vi "LCP Set Volume Unit.vi"(7 "Prefix":T2=-3 items=["UNIT"=0, "DECI"=-1, "CENTI"=-2, "MILLI"=-3, "MICRO"=-6], 8 "error in (no error)":errorcluster caption="Fehler (Eingang, kein Fehler)", 10 "Volume Unit":T1 items=["LITRES"=68], 11 "Pump Handle":i64) -> (0 "error out":errorcluster caption="Fehler (Ausgang)")   [LabVIEW 2023, in "labbCAN_Pump_API.lvlib"]
doc: "LCP_Func long LCP_CALL LCP_SetVolumeUnit(dev_hdl hPump,\n int Prefix,\n int VolumeUnit);"
uses:
  labbCAN_Pump_API.lvlib
  labbCAN_Bus_API/SiUnitPrefix.ctl
  VolumeUnits.ctl
  labbCAN_Pump_API.dll
  labbCAN_Bus_API/labbCAN_Bus_API.lvlib
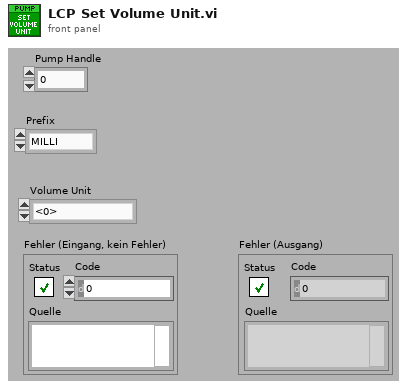
[diagram p1: front panel]
types:
  T1 = typedef "labbCAN_Pump_API.lvlib/VolumeUnits.ctl" = i32
  T2 = typedef "labbCAN_Bus_API.lvlib/SiUnitPrefix.ctl" = i32
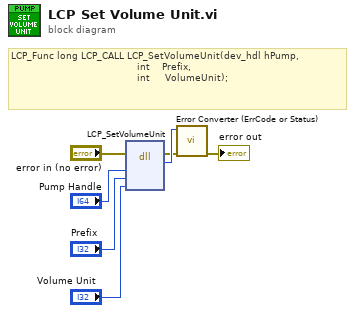
[diagram p0: block diagram]
diagram:
  # "LCP_Func long LCP_CALL LCP_SetVolumeUnit(dev_hdl hPump,\n                                          int    Prefix,\n                                          int     VolumeUnit);"
  n1 = dll-call lib="C:/GIT/DensityGradientProject/CETONI_SDK/labbCAN_Pump_API.*" fn="LCP_SetVolumeUnit"(error in="error in (no error)", "hPump"="Pump Handle", "Prefix"="Prefix", "VolumeUnit"="Volume Unit") -> (error out=w2:errorcluster, "Rückgabetyp"=w3:i32)  [unwired: 5 in, 1 out]
  n2 = call "Error Converter (ErrCode or Status).vi"("error in (no error)"=w2, "error code"=w3) -> ("error out"=→"error out":errorcluster)  [unwired: 9 in]
